vi "Action Update Heater State.vi"(8 "error in (no error)":errorcluster, 9 "Heater State":T1, 10 "Temperature Ramp Rate":dbl, 11 "Temperature Set Point":dbl) -> (0 "error out":errorcluster)   [LabVIEW 2018, in "Thermal Chamber Controller_DQMH.lvlib"]
uses:
  Thermal Chamber Controller_DQMH.lvlib
  Heater State--enum.ctl
  Thermal Chamber Response Simulator/Thermal Chamber Response Simulator.lvlib
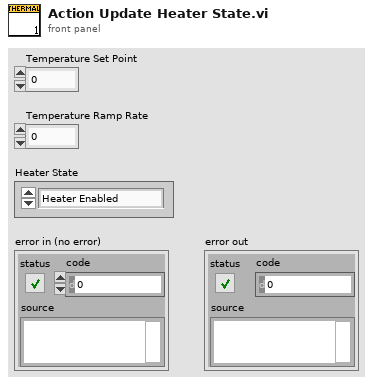
[diagram p1: front panel]
types:
  T1 = typedef "Thermal Chamber Controller_DQMH.lvlib/Heater State--enum.ctl" = enum16{"Heater Enabled", "Heater Disabled"}
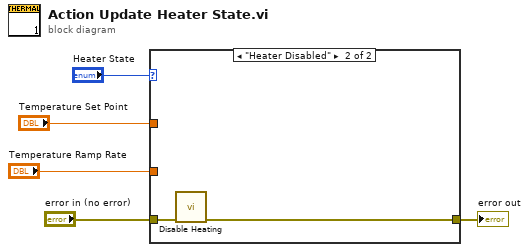
[diagram p0: block diagram]
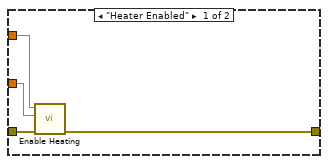
[diagram p2: hidden frame]
diagram:
  n1 = case shown="\"Heater Disabled\"" "Heater State" {
    tunnel: "error in (no error)" -> [w9 w11]
    tunnel: [w8 w10] -> w1
    tunnel: "Temperature Set Point" -> [w6 _]
    tunnel: "Temperature Ramp Rate" -> [w7 _]
    frame "Heater Enabled" {
      n2 = call "Enable Heating.vi"("error in (no error)"=w9, "Ramp Rate (deg C / second)"=w7, "Temperature Set Point (deg C)"=w6) -> ("error out"=w8:errorcluster)  [unwired: 8 in]
    }
    frame "Heater Disabled" {
      n3 = call "Disable Heating.vi"("error in (no error)"=w11) -> ("error out"=w10:errorcluster)  [unwired: 10 in]
    }
  }
  "error out" <- w1
